vi "OFDMRx2.vi"(0 "Input Signal":cdb[](array[numeric]), 1 "Frequency Offset":dbl format="%#_13g", 2 "Channel Taps":dbl[](array[numeric]), 3 "Equalize":bool, 4 "Transmitter Properties":T1 {"Window" items=["Rectangular", "Bohman", "Parzen", "Bartlett-Hanning", "Blackman-Nuttall", "Blackman", "Hanning", "Hamming", "Welch", "Exact Blackman", "Blackman-Harris", "Triangle"]}) -> (5 "Output Bits":bool[](array[boolean]))   [LabVIEW 2013]
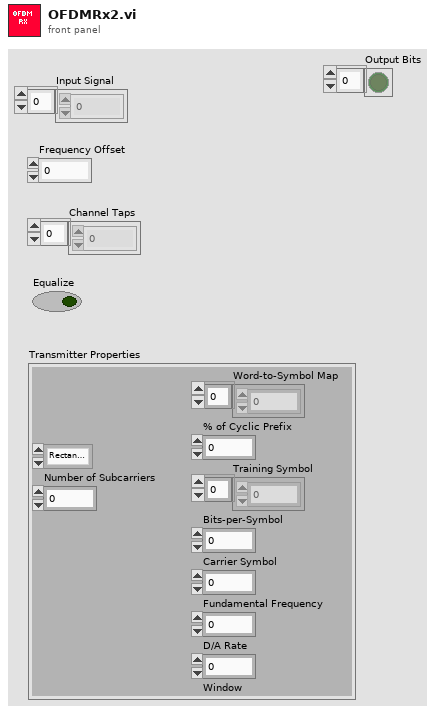
[diagram p1: front panel]
types:
  T1 = cluster{"Word-to-Symbol Map":cdb[], "% of Cyclic Prefix":dbl, "Training Symbol":cdb[], "Bits-per-Symbol":i32, "Carrier Symbol":cdb, "Fundamental Frequency":dbl, "D/A Rate":dbl, "Window":u16, "Number of Subcarriers":i32}
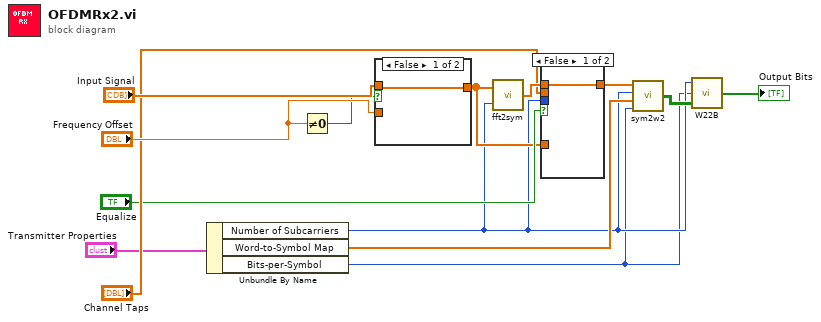
[diagram p0: block diagram]
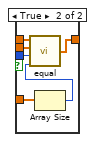
[diagram p2: hidden frame]
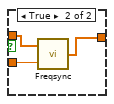
[diagram p3: hidden frame]
diagram:
  n1 = Unbundle By Name("Transmitter Properties") -> ("Number of Subcarriers"=w2:i32, "Word-to-Symbol Map"=w3:cdb[], "Bits-per-Symbol"=w1:i32)
  n2 = Not Equal To 0?(x="Frequency Offset") -> (x != 0?=w12:bool)
  n3 = case shown="False" w12 {
    tunnel: "Input Signal" -> [w15 w18]
    tunnel: "Frequency Offset" -> [_ w17]
    tunnel: [w15 w16] -> w7
    frame False {
    }
    frame True {
      n4 = call "Freqsync.vi"("Frequency Offset"=w17, "Offset Signal 2"=w18) -> ("Corrected Signal 2"=w16:cdb[])
    }
  }
  n5 = call "fft2sym.vi"("Number of Subcarriers"=w2, "Time domain In"=w7) -> ("Parallel Symbole out 2"=w11:cdb[])
  n6 = case shown="False" "Equalize" {
    tunnel: w11 -> [w19 w25]
    tunnel: "Channel Taps" -> [_ w24]
    tunnel: [w19 w21] -> w9
    tunnel: w7 -> [_ w23]
    tunnel: w2 -> [_ w20]
    frame False {
    }
    frame True {
      n7 = Array Size(array=w23) -> (size(s)=w22:i32)
      n8 = call "equal.vi"("Symbol Size"=w22, "Number of Subcarriers"=w20, "Channel Taps"=w24, "Unequalized Signal"=w25) -> ("Equalized Signal"=w21:cdb[])
    }
  }
  n9 = call "sym2w2.vi"("Bits-per-Symbol"=w1, "Word-to-Symbol Map 2"=w3, "Number of Subcarriers"=w2, "Parallel Symbol input"=w9) -> ("Parallel Word Output"=w6:bool[][])
  n10 = call "W22B.vi"("Parallel Word In"=w6, "Bits-per-Symbol"=w1, "Number of Subcarries"=w2) -> ("Parallel Output"=→"Output Bits":bool[])
